vi "NI VeriStand - Close Calibration Reference.vi"(8 "error in":errorcluster, 11 "Calibration":T1) -> (0 "error out":errorcluster)   [LabVIEW 2020, in "NI_VS Calibration ExecutionAPI.lvlib"]
doc: "Closes an open reference to the calibration tool on the VeriStand Gateway. Use this VI to close each calibration manager reference that you open with the Open Calibration Reference VI."
uses:
  <vilib>/NI VeriStand/Execution/Calibration/NI_VS Calibration ExecutionAPI.lvlib
  <vilib>/NI VeriStand/Execution/Calibration/CalibrationAPI.ctl
  NationalInstruments.VeriStand.ClientAPI
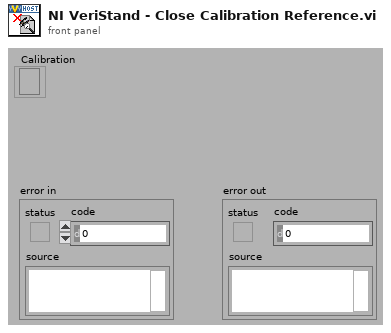
[diagram p1: front panel]
types:
  T1 = typedef "NI_VS Calibration ExecutionAPI.lvlib/CalibrationAPI.ctl" = refnum<k24>
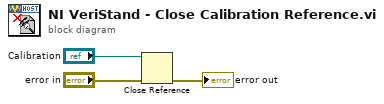
[diagram p0: block diagram]
diagram:
  n1 = Close Reference(reference="Calibration", error in (no error)="error in") -> (error out=→"error out":errorcluster)
